vi "Get ROI Grid Definition.vi"(8 "error in (no error)":errorcluster, 10 "Current ROI Bounds":T1, 11 "Enable":bool=TRUE) -> (0 "error out":errorcluster, 1 "OK":bool, 2 "ROI Bounds out":T1, 3 "Grid Definition":T2)   [LabVIEW 2021, in "Image.lvlib"]
uses:
  Image.lvlib
  ROI Grid Definition.ctl
  ROI  Type.ctl
  ROI Bounds.ctl
panel:
  in  "Grid Definition":T2
  out "String":string
  in  "Cancel":bool
  in  "OK2":bool
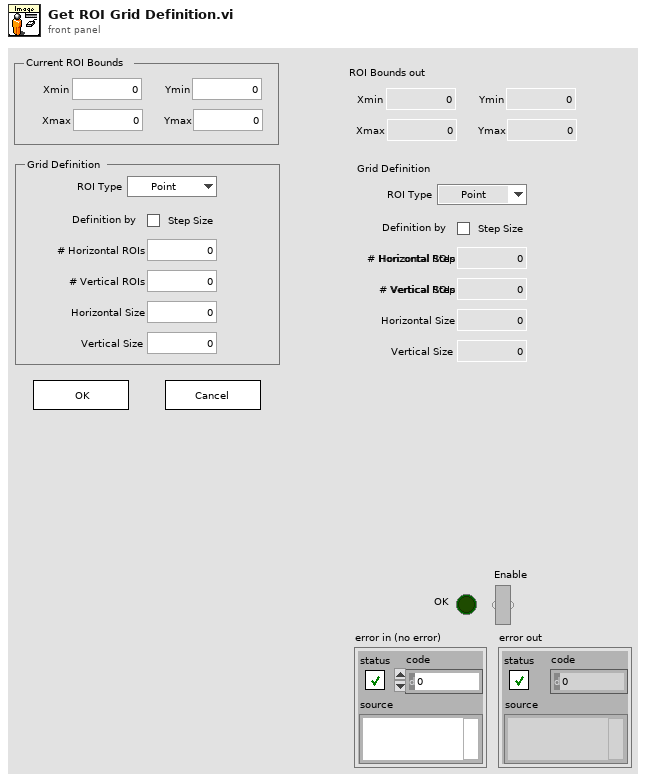
[diagram p1: front panel]
types:
  T1 = typedef "Image.lvlib/ROI Bounds.ctl" = cluster{"Ymax":i32, "Xmin":i32, "Ymin":i32, "Xmax":i32}
  T2 = typedef "Image.lvlib/ROI Grid Definition.ctl" = cluster{"Horizontal Step":i32, "Vertical Step":i32, "Horizontal Size":i32, "Vertical Size":i32, "# Horizontal ROIs":i32, "# Vertical ROIs":i32, "Definition by":bool, "ROI Type":T3}
  T3 = typedef "Image.lvlib/ROI  Type.ctl" = enum16{"Point", "Oval", "Rectangle"}
  T4 = cluster{"Input Name":string, "Input Data Type":i32}[]
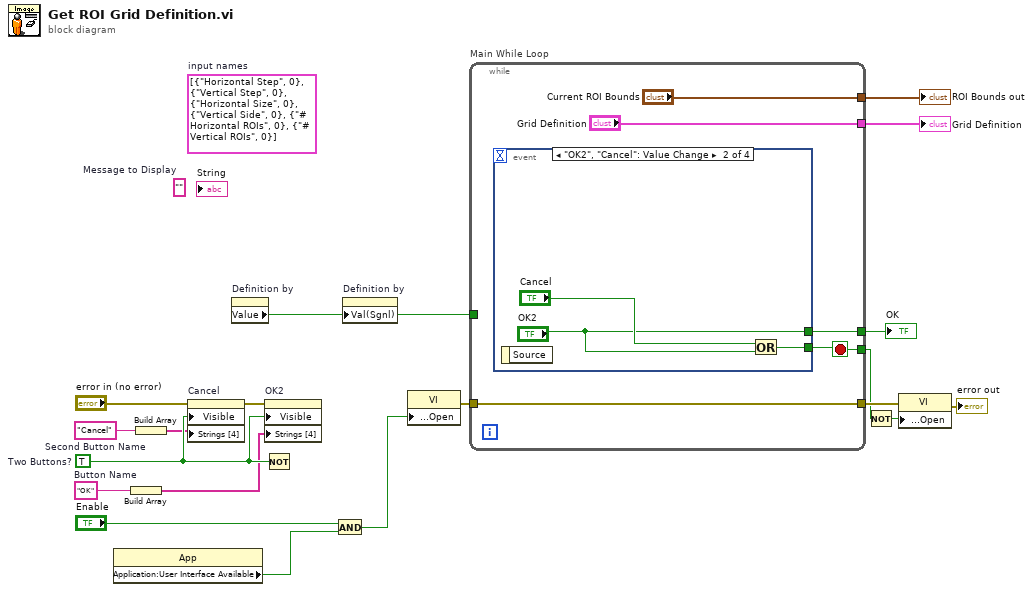
[diagram p0: block diagram]
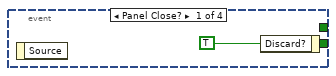
[diagram p2: hidden frame]
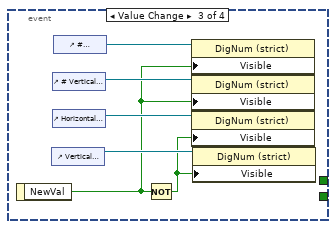
[diagram p3: hidden frame]
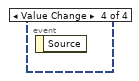
[diagram p4: hidden frame]
diagram:
  (unwired) T4 [{"Input Name"="Horizontal Step", "Input Data Type"=0}, {"Input Name"="Vertical Step", "Input Data Type"=0}, {"Input Name"="Horizontal Size", "Input Data Type"=0}, {"Input Name"="Vertical Side", "Input Data Type"=0}, {"Input Name"="# Horizontal ROIs", "Input Data Type"=0}, {"Input Name"="# Vertical ROIs", "Input Data Type"=0}]  # input names
  w15 = "Cancel"  # Second Button Name
  w13 = "OK"  # Button Name
  (unwired) ""  # Message to Display
  w19 = TRUE  # Two Buttons?
  n1 = property class="App"() -> ("Application:User Interface Available"=w6:bool)  [unwired: 2 in, 2 out]
  n2 = Build Array(w13) -> (w14:string[])
  n3 = Build Array(w15) -> (w16:string[])
  n4 = property on="Cancel" class="Bool"(error in="error in (no error)", "Visible"=w19, "Strings [4]"=w16) -> (error out=w18:errorcluster)  [unwired: 1 in, 1 out]
  n5 = property on="Definition by" class="Bool (strict)"() -> ("Value"=w5:bool)  [unwired: 2 in, 2 out]
  n6 = Not(x=w19) -> ()  [unwired: 1 out]
  n7 = property on="OK2" class="Bool"(error in=w18, "Visible"=w19, "Strings [4]"=w14) -> ()  [unwired: 1 in, 2 out]
  n8 = And(x="Enable", y=w6) -> (x .and. y?=w7:bool)
  n9 = property on="Definition by" class="Bool (strict)"("Val(Sgnl)"=w5) -> ()  [unwired: 2 in, 2 out]
  n10 = property class="VI"("Front Panel Window:Open"=w7) -> (error out=w12:errorcluster)  [unwired: 2 in, 1 out]
  n11 = while "Main While Loop" {
    tunnel: w12 -> [w24]
    tunnel: [w24] -> w10
    tunnel: w5 -> [_]
    tunnel: [w23] -> w4
    tunnel: [w22] -> w3
    tunnel: ["Grid Definition"] -> w2
    tunnel: ["Current ROI Bounds"] -> w1
    stop <- w22 stop-if-true
    n12 = event shown="[1] \"OK2\", \"Cancel\": Value Change" {
      selector: _ -> [_ _ _ _]
      dyn-events: _ -> [_ _ _ _]
      timeout: _ -> [_ _ _ _]
      tunnel: [w25 w27 _ _] -> w22
      tunnel: [_ "OK2" _ _] -> w23
      event Panel Close? {
        w25 = TRUE ("Discard?")
        n13 = event-data() -> ()  [unwired: 1 in, 1 out]
        n14 = event-data("Discard?"=w25) -> ()  [unwired: 1 in, 1 out]
      }
      event "OK2", "Cancel": Value Change {
        n15 = event-data() -> ()  [unwired: 1 in, 1 out]
        n16 = Or(x="Cancel", y="OK2") -> (x .or. y?=w27:bool)
      }
      event Value Change {
        n17 = event-data() -> ("NewVal"=w30:bool)  [unwired: 1 in]
        n18 = control-ref of="Vertical Step"() -> (w31:refnum<vi>)
        n19 = control-ref of="# Vertical ROIs"() -> (w33:refnum<vi>)
        n20 = control-ref of="Horizontal Step"() -> (w32:refnum<vi>)
        n21 = control-ref of="# Horizontal ROIs"() -> (w34:refnum<vi>)
        n22 = Not(x=w30) -> (.not. x?=w29:bool)
        n23 = property class="DigNum (strict)"(reference=w34, "Visible"=w30) -> ()  [unwired: 1 in, 2 out]
        n24 = property class="DigNum (strict)"(reference=w33, "Visible"=w30) -> ()  [unwired: 1 in, 2 out]
        n25 = property class="DigNum (strict)"(reference=w32, "Visible"=w29) -> ()  [unwired: 1 in, 2 out]
        n26 = property class="DigNum (strict)"(reference=w31, "Visible"=w29) -> ()  [unwired: 1 in, 2 out]
      }
      event Value Change {
        n27 = event-data() -> ()  [unwired: 1 in, 1 out]
      }
    }
  }
  "OK" <- w4
  "Grid Definition" <- w2
  "ROI Bounds out" <- w1
  n28 = Not(x=w3) -> (.not. x?=w17:bool)
  n29 = property class="VI"(error in=w10, "Front Panel Window:Open"=w17) -> (error out=→"error out":errorcluster)  [unwired: 1 in, 1 out]
